vi "setReadingTime.vi"(8 "error in (no error)":errorcluster, 10 "Period":T1, 11 "ElectrometerController in":refnum<class "ElectrometerController.lvclass">) -> (0 "error out":errorcluster, 3 "ElectrometerController out":refnum<class "ElectrometerController.lvclass">)   [LabVIEW 2016, in "ElectrometerController.lvclass"]
uses:
  ElectrometerController.lvclass
  ts_electrometeruserevents/Typedefs/MeasuringPeriod.ctl
  ElectrometerController.lvclass/ElectrometerController.ctl
  ts_electrometeruserevents/MiddlewareSALThisComponent/MiddlewareSALThisComponent.lvclass
  ts_electrometeruserevents/Typedefs/ElectrometerTypedefs.lvlib
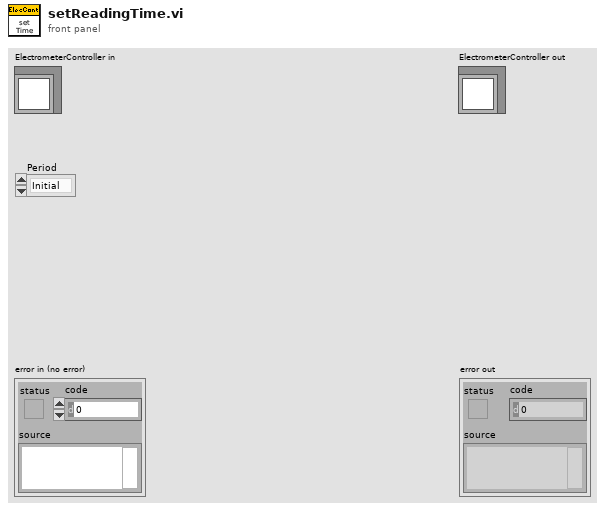
[diagram p1: front panel]
types:
  T1 = typedef "ElectrometerTypedefs.lvlib/MeasuringPeriod.ctl" = enum16{"Initial", "End"}
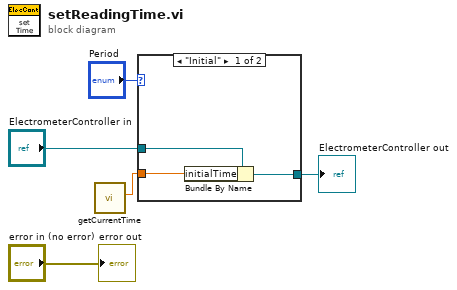
[diagram p0: block diagram]
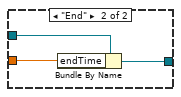
[diagram p2: hidden frame]
diagram:
  n1 = call "getCurrentTime.vi"() -> ("timestamp"=w3:dbl)  [unwired: 9 in, 2 out]
  n2 = case shown="\"Initial\"" "Period" {
    tunnel: w3 -> [w6 w9]
    tunnel: "ElectrometerController in" -> [w8 w11]
    tunnel: [w7 w10] -> w2
    frame "Initial" {
      n3 = Bundle By Name(cluster=w8, "initialTime"=w6) -> (w7:refnum<class "ElectrometerController.lvclass">)
    }
    frame "End" {
      n4 = Bundle By Name(cluster=w11, "endTime"=w9) -> (w10:refnum<class "ElectrometerController.lvclass">)
    }
  }
  "ElectrometerController out" <- w2
  "error out" <- "error in (no error)"
